vi "Read Program Status.vi"(7 "Unit Address (1)":u8=1, 8 "error in (no error)":errorcluster, 11 "VISA resource name":refnum<visa-resource-name>) -> (0 "error out":errorcluster, 1 "Program Status\n- Array of Bits":bool[](array[boolean]), 2 "Program Status\n- Decimal":u16(ring)=1 items=["Off"=1, "Run"=2, "Hold"=4, "Holdback"=8, "Complete"=16], 3 "VISA resource name out":refnum<visa-resource-name>)   [LabVIEW 2014, in "Eurotherm 35xx Series.lvlib"]
doc: "This VI returns Program Status."
uses:
  <instrlib>/Eurotherm 35xx Series/Eurotherm 35xx Series.lvlib
panel:
  # "Bit 0"
  # "Off"
  # "Bit 1"
  # "Run"
  # "Bit 2"
  # "Hold"
  # "Bit 3"
  # "Holdback"
  # "Bit 4"
  # "Complete"
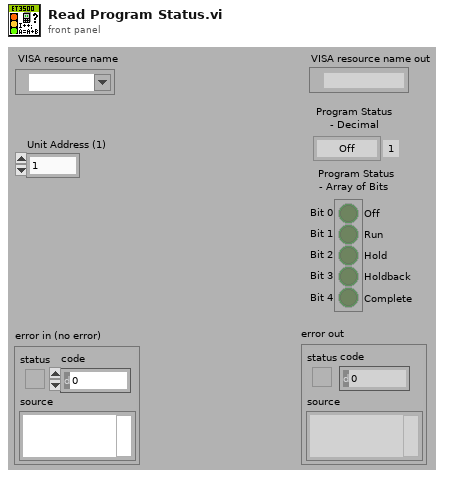
[diagram p1: front panel]
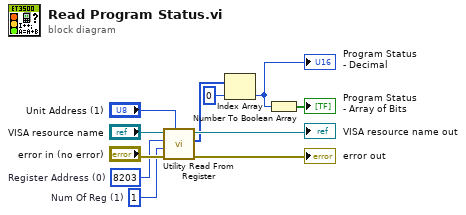
[diagram p0: block diagram]
diagram:
  w3 = u16 8203  # Register Address (0)
  w7 = u16 1  # Num Of Reg (1)
  n1 = call <instrlib>:"Utility Read From Register.vi"("Unit Address (1)"="Unit Address (1)", "error in (no error)"="error in (no error)", "Num Of Reg (1)"=w7, "Register Address (0)"=w3, "VISA resource name"="VISA resource name") -> ("error out"=→"error out":errorcluster, "Data"=w5:i16[], "VISA resource name out"=→"VISA resource name out":refnum<visa-resource-name>)  [unwired: 4 in]
  n2 = Index Array(array=w5, index=0) -> (element=w2:i16)
  "Program Status\n- Decimal" <- w2
  n3 = Number To Boolean Array(number=w2) -> (Boolean array=→"Program Status\n- Array of Bits":bool[])
